vi "Read FileProperties.vi"(8 "error in (no error)":errorcluster, 10 "Read":bool, 11 "Path in":refnum<vi>) -> (0 "error out":errorcluster, 2 "File Properties":T1, 3 "VI out":refnum<vi>)   [LabVIEW 2020]
uses:
  TDefs/Single File Properties.ctl
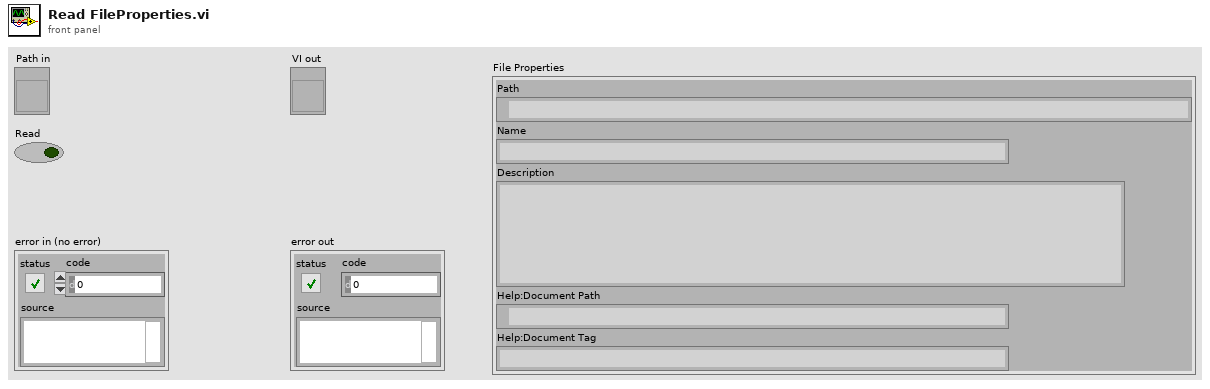
[diagram p1: front panel]
types:
  T1 = typedef "Single File Properties.ctl" = cluster{"Path":path, "Name":string, "Description":string, "Help:Document Path":path, "Help:Document Tag":string}
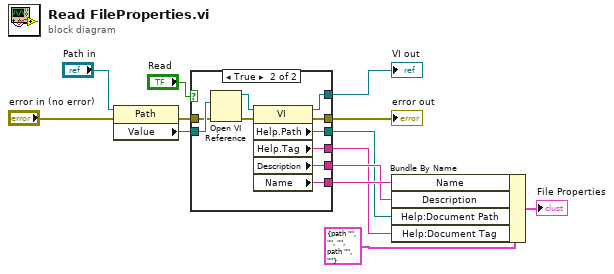
[diagram p0: block diagram]
diagram:
  n1 = property on="Property Node" class="Path"(reference="Path in", error in="error in (no error)") -> (error out=w10:errorcluster, "Value"=w11:path)  [unwired: 1 out]
  n2 = case shown="True" "Read" {
    tunnel: [_ w24] -> w3
    tunnel: [_ w23] -> w2
    tunnel: [_ w22] -> w4
    tunnel: [_ w21] -> w5
    tunnel: w10 -> [w14 w17]
    tunnel: [w14 w20] -> w13
    tunnel: w11 -> [_ w18]
    tunnel: [_ w15] -> w12
    frame False {
    }
    frame True {
      n3 = Open VI Reference(vi path=w18, error in (no error)=w17) -> (vi reference=w19:refnum<vi>, error out=w16:errorcluster)  [unwired: 4 in]
      n4 = property class="VI"(reference=w19, error in=w16) -> (reference out=w15:refnum<vi>, error out=w20:errorcluster, "Help.Path"=w24:path, "Help.Tag"=w23:string, "Description"=w22:string, "Name"=w21:string)
    }
  }
  "error out" <- w13
  "VI out" <- w12
  n5 = Bundle By Name(cluster=T1 {"Path"=path "", "Name"="", "Description"="", "Help:Document Path"=path "", "Help:Document Tag"=""} ("File Properties"), "Name"=w5, "Description"=w4, "Help:Document Path"=w3, "Help:Document Tag"=w2) -> (→"File Properties":T1)
